vi "Write Selector.vi"(5 "Selector":refnum<class "Tunnel.lvclass">, 9 "CaseStructure in":refnum<class "CaseStructure.lvclass">) -> (3 "CaseStructure out":refnum<class "CaseStructure.lvclass">)   [LabVIEW 2014, in "CaseStructure.lvclass"]
uses:
  CaseStructure.lvclass
  Tunnel/Tunnel.lvclass
  CaseStructure.lvclass/CaseStructure.ctl
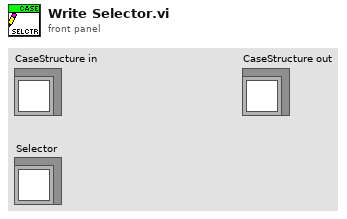
[diagram p1: front panel]
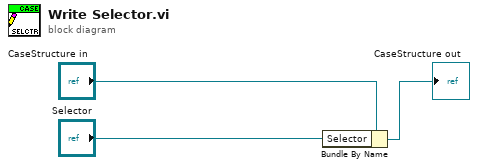
[diagram p0: block diagram]
diagram:
  n1 = Bundle By Name(cluster="CaseStructure in", "Selector"="Selector") -> (→"CaseStructure out":refnum<class "CaseStructure.lvclass">)
